vi "Number_Of_Rotations.vi"(10 "No of Slits":dbl, 11 "Encoder Count":dbl) -> (3 "Number Of Rotations":dbl)   [LabVIEW 2018]
doc: "This VI calculates current number of rotations by dividing current counter value by the number of slits on the encoder wheel (4).\n\nInputs:\nEncoder count;\nNo of slits.\n\nOutputs:\nNumber of rotations."
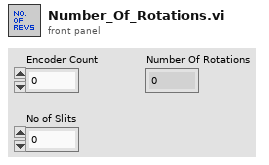
[diagram p1: front panel]
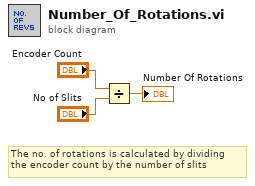
[diagram p0: block diagram]
diagram:
  # "The no. of rotations is calculated by dividing\nthe encoder count by the number of slits"
  n1 = Divide(x="Encoder Count", y="No of Slits") -> (x/y=→"Number Of Rotations":dbl)
